vi "XML Parse String Range.vi"(3 "Attribut Name":string, 7 "XML Response":string, 8 "Anzahl Elemente":i32) -> (0 "Elemente (Strings)":string[](array[string]), 2 "XML Response gekürzt":string)   [LabVIEW 2020, in "FT-IR.lvlib" / "TOOLweb Interface.lvlib" / "TOOLweb Interface Hilfs-VIs.lvlib"]
doc: "Sucht in dem XML-Poll-Response-String \"XML-Response\" den Eintrag mit dem Elementnamen \"Attribut Name\" und liefert dessen Werte im String-Array \"Elemente (Strings)\". \n\nDer Eintrag wird dann entfernt, damit eine weiteres Parser-VI am Ausgang \"XML Response gekürzt\" nicht wieder den ganzen String durchsuchen muss."
uses:
  TOOLweb Interface Hilfs-VIs.lvlib
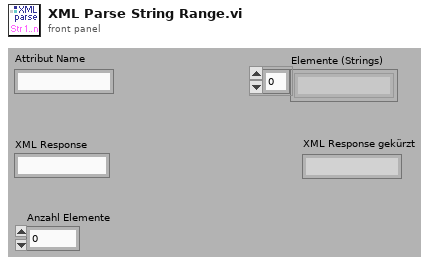
[diagram p1: front panel]
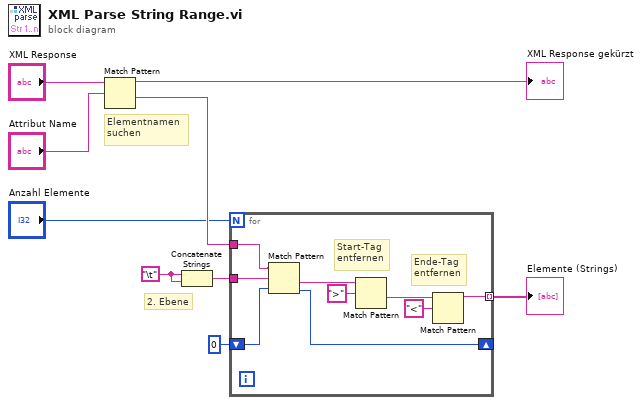
[diagram p0: block diagram]
diagram:
  w6 = "\t"
  # "2. Ebene"
  # "Elementnamen\nsuchen"
  n1 = Match Pattern(string="XML Response", regular expression="Attribut Name") -> (before substring=→"XML Response gekürzt":string, after substring=w3:string)  [unwired: 3 out]
  n2 = Concatenate Strings(w6, w6) -> (w5:string)
  n3 = for {
    N: "Anzahl Elemente" -> [_]
    tunnel: w3 -> [w18]
    tunnel: w5 -> [w17]
    shift-right: [w15] -> _
    shift-left: 0 ("offset past match") -> [w16]
    tunnel: [w10] -> w1 mode=indexing
    # "Start-Tag\nentfernen"
    # "Ende-Tag\nentfernen"
    n4 = Match Pattern(string=w18, regular expression=w17, offset (0)=w16) -> (after substring=w14:string, offset past match=w15:i32)  [unwired: 2 out]
    n5 = Match Pattern(string=w14, regular expression=">" ("Regulärer Ausdruck")) -> (after substring=w11:string)  [unwired: 4 out]
    n6 = Match Pattern(string=w11, regular expression="<" ("Regulärer Ausdruck")) -> (before substring=w10:string)  [unwired: 4 out]
  }
  "Elemente (Strings)" <- w1
